vi "Override Target Timing Source.vi"(8 "error in (no error)":errorcluster, 11 "CD Ref in":T1 format="%.0x") -> (0 "error out":errorcluster, 3 "CD Ref out":T1 format="%.0x")   [LabVIEW 2019, in "TimingDRV System Explorer.lvlib"]
uses:
  TimingDRV System Explorer.lvlib
  <vilib>/NI VeriStand/Custom Device API/Custom Device Item Ref.ctl
  NationalInstruments.VeriStand.SystemDefinitionAPI
  NationalInstruments.VeriStand.SystemStorage
  <vilib>/NI VeriStand/Custom Device Tools/Custom Device Utility Library/Custom Device Utility Library.lvlib
  <vilib>/NI VeriStand/Custom Device API/Custom Device API.lvlib
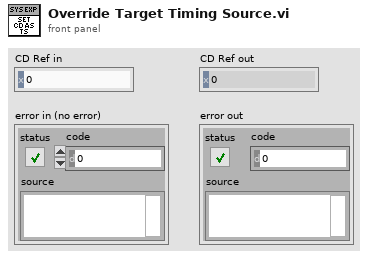
[diagram p1: front panel]
types:
  T1 = typedef "Custom Device API.lvlib/Custom Device Item Ref.ctl" = u64
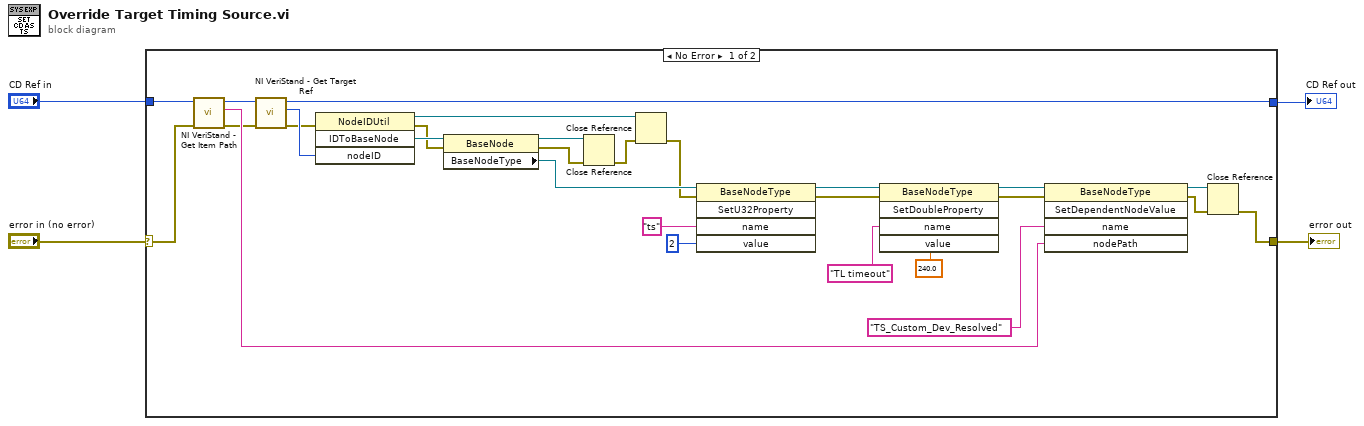
[diagram p0: block diagram]
diagram:
  n1 = case shown="No Error" "error in (no error)" {
    selector: "error in (no error)" -> [w7 w34]
    tunnel: [w8 w33] -> w4
    tunnel: [w9 w34] -> w3
    tunnel: "CD Ref in" -> [w10 w33]
    frame No Error {
      n2 = call <vilib>:"NI VeriStand - Get Item Path.vi"("error in (no error)"=w7, "Item Ref in"=w10) -> ("error out"=w16:errorcluster, "Path"=w18:string, "Item Ref out"=w17:T1)  [unwired: 6 in, 1 out]
      n3 = call <vilib>:"NI VeriStand - Get Target Ref.vi"("error in"=w16, "Item Ref in"=w17) -> ("error out"=w29:errorcluster, "Target Ref"=w32:T1, "Item Ref out"=w8:T1)  [unwired: 6 in, 1 out]
      n4 = invoke class="NodeIDUtil" method="IDToBaseNode"(error in=w29, "nodeID"=w32) -> (reference out=w26:refnum<k24>, error out=w27:errorcluster, "IDToBaseNode"=w28:refnum<k24>)  [unwired: 2 in, 1 out]
      n5 = property class="BaseNode"(reference=w28, error in=w27) -> (reference out=w24:refnum<k24>, error out=w25:errorcluster, "BaseNodeType"=w31:refnum<k24>)
      n6 = Close Reference(reference=w24, error in (no error)=w25) -> (error out=w23:errorcluster)
      n7 = Close Reference(reference=w26, error in (no error)=w23) -> (error out=w30:errorcluster)
      n8 = invoke class="BaseNodeType" method="SetU32Property"(reference=w31, error in=w30, "name"="ts", "value"=u32 2) -> (reference out=w20:refnum<k24>, error out=w19:errorcluster)  [unwired: 1 in, 3 out]
      n9 = invoke class="BaseNodeType" method="SetDoubleProperty"(reference=w20, error in=w19, "name"="TL timeout", "value"=240.0) -> (reference out=w21:refnum<k24>, error out=w22:errorcluster)  [unwired: 1 in, 3 out]
      n10 = invoke class="BaseNodeType" method="SetDependentNodeValue"(reference=w21, error in=w22, "name"="TS_Custom_Dev_Resolved", "nodePath"=w18) -> (reference out=w5:refnum<k24>, error out=w6:errorcluster)  [unwired: 1 in, 3 out]
      n11 = Close Reference(reference=w5, error in (no error)=w6) -> (error out=w9:errorcluster)
    }
    frame Error {
    }
  }
  "CD Ref out" <- w4
  "error out" <- w3
